vi "读MCDS参数设置.vi"() -> ()   [LabVIEW 2010]
uses:
  <vilib>/Utility/file.llb/Write To Spreadsheet File (string).vi
  GlobalVariable.vi
panel:
  out "选定曲线信息":string[](array[string])
  in  "曲线显示开关":bool[](array[boolean])
  in  "地址":sgl[][](array[numeric])
  in  "附加10点地址":i32=4
  in  "TCP 端口":i32=4
  in  "报警限值":sgl
  in  "报警延时":i32
  in  "报警点地址":i32
  in  "写寄存器数量":i32=4
  in  "写寄存器开始地址":i32=4
  in  "读寄存器数量":i32=4
  in  "读寄存器开始地址":i32=4
  in  "下段文件浏览":bool
  in  "上段文件浏览":bool
  in  "TCP IP地址":string
  in  "USB虚拟串口":string
  in  "取消修改":bool caption="Cancel Button"
  in  "保存修改":bool
  # "读取MCDS网络参数设置"
  # "坐标MAX"
  # "坐标MIN"
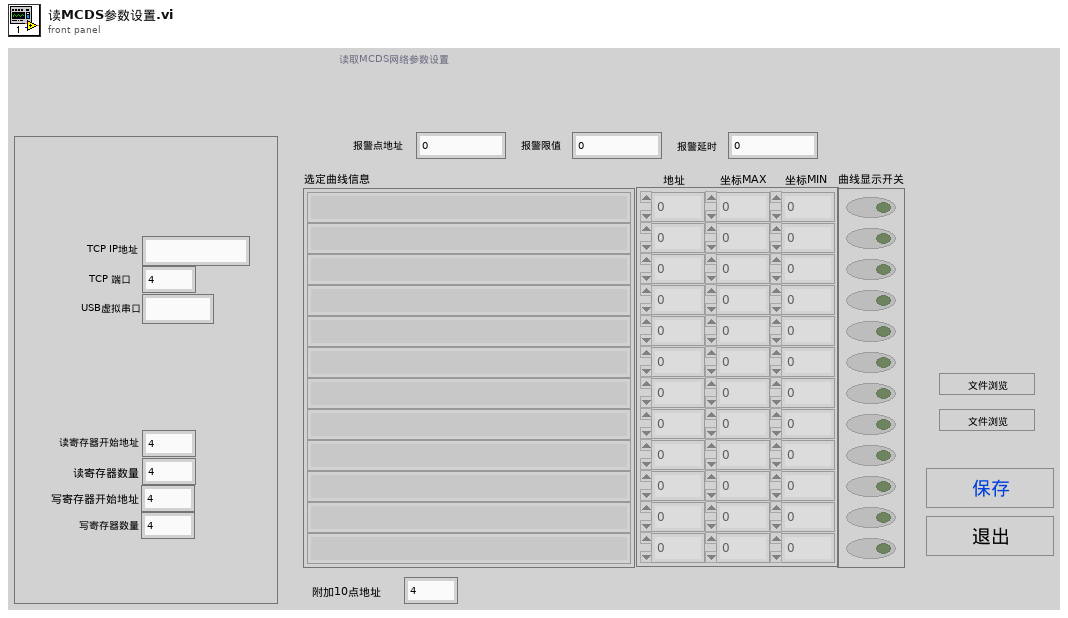
[diagram p1: front panel]
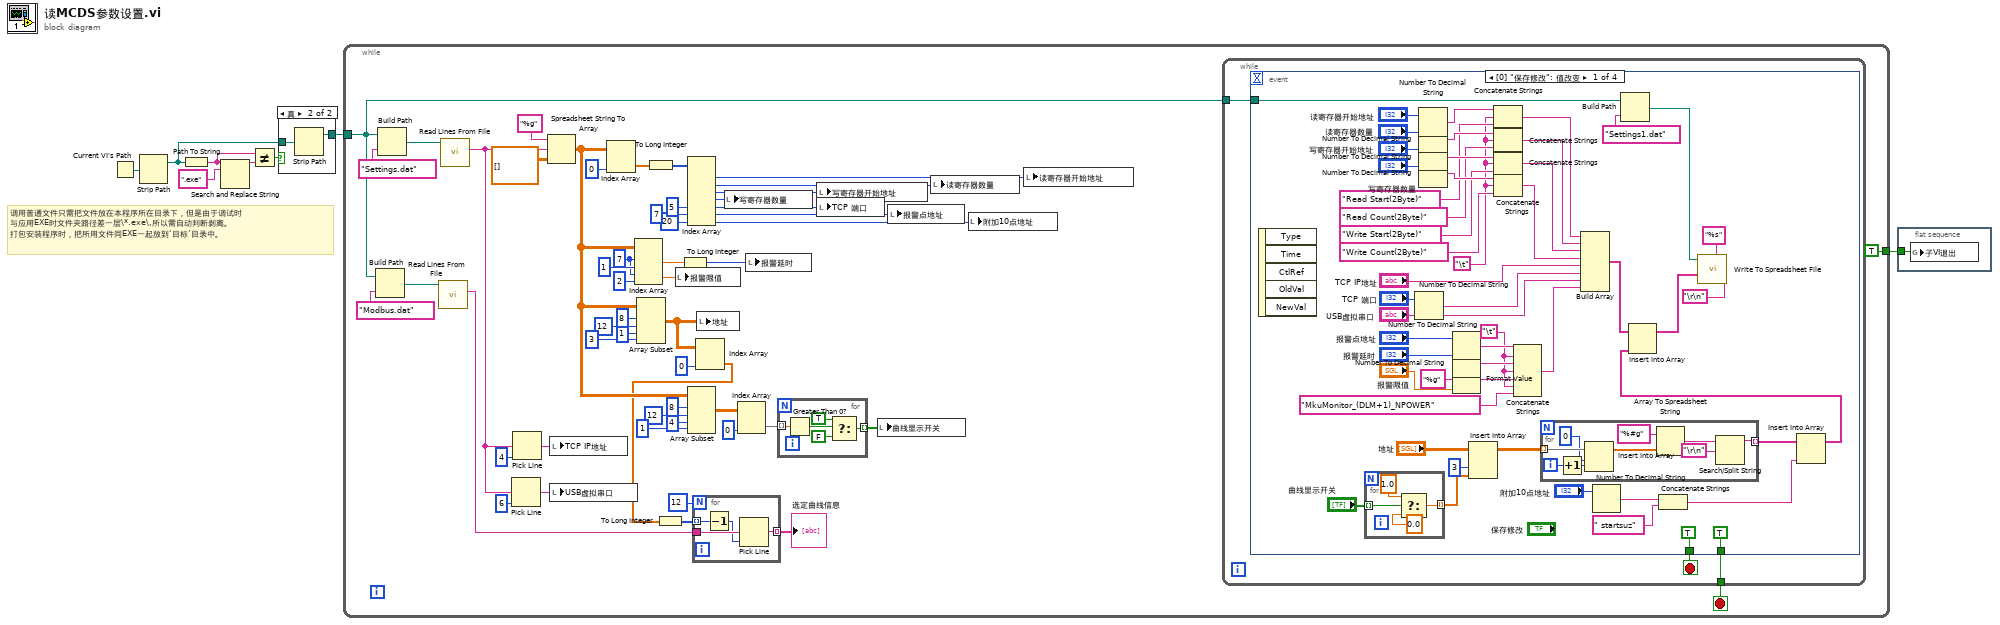
[diagram p0: block diagram]
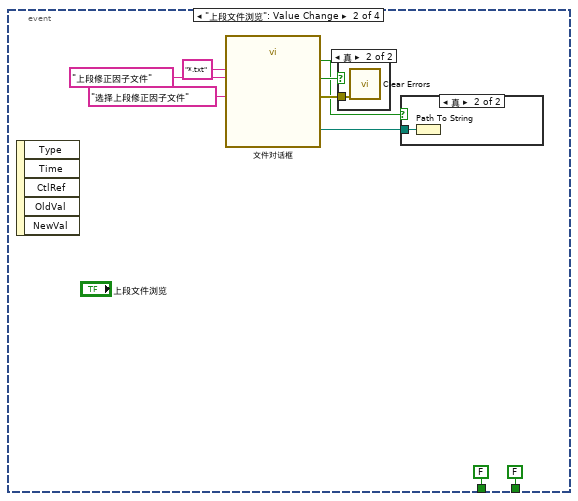
[diagram p3: hidden frame]
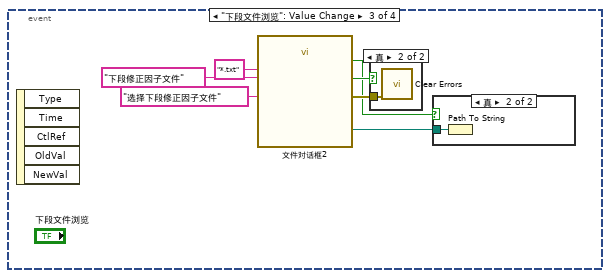
[diagram p6: hidden frame]
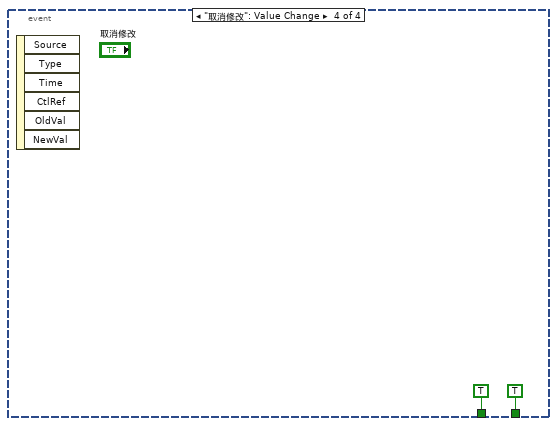
[diagram p9: hidden frame]
diagram:
  # "调用普通文件只需把文件放在本程序所在目录下，但是由于调试时\n与应用EXE时文件夹路径差一层\\*.exe\\,所以需自动判断剥离。\n打包安装程序时，把所用文件同EXE一起放到‘目标’目录中。"
  n1 = Current VI's Path() -> (path=w3:path)
  n2 = Strip Path(path=w3) -> (stripped path=w8:path)  [unwired: 1 out]
  n3 = Path To String(path=w8) -> (string=w6:string)
  n4 = Search and Replace String(input string=w6, search string=".exe" ("搜索字符串")) -> (result string=w5:string)  [unwired: 6 in, 3 out]
  n5 = Not Equal?(x=w6, y=w5) -> (x != y?=w7:bool)
  n6 = case shown="真" w7 {
    tunnel: w8 -> [w9 w11]
    tunnel: [w9 w10] -> w2
    frame False {
    }
    frame True {
      n7 = Strip Path(path=w11) -> (stripped path=w10:path)  [unwired: 1 out]
    }
  }
  n8 = while {
    tunnel: w2 -> [w12]
    tunnel: [TRUE ("子VI退出")] -> w1
    stop <- w63 stop-if-true
    w39 = 7 ("索引 (行)")
    n9 = Build Path(base path=w12, name or relative path="Modbus.dat") -> (appended path=w20:path)
    n10 = Build Path(base path=w12, name or relative path="Settings.dat") -> (appended path=w61:path)
    n11 = call <vilib>:"Read Lines From File.vi"("file path (dialog if empty)"=w20) -> ("line string"=w19:string)  [unwired: 5 in, 3 out]
    n12 = call <vilib>:"Read Lines From File.vi"("file path (dialog if empty)"=w61) -> ("line string"=w52:string)  [unwired: 5 in, 3 out]
    n13 = Pick Line ("选行并添加至字符串")(multi-line string=w52, line index=6 ("行索引")) -> (output string=w51:string)  [unwired: 1 in]
    n14 = Pick Line ("选行并添加至字符串")(multi-line string=w52, line index=4 ("行索引")) -> (output string=w54:string)  [unwired: 1 in]
    n15 = Spreadsheet String To Array ("电子表格字符串至数组转换")(format string="%g" ("format (%.3f)"), spreadsheet string=w52, array type (2D Dbl)=sgl[][] [] ("数组类型(2D Dbl)")) -> (array=w26:sgl[][])  [unwired: 1 in]
    n16 = local write "TCP IP地址"(w54) -> ()
    n17 = local write "USB虚拟串口"(w51) -> ()
    n18 = Index Array(array=w26, index (col)=0 ("禁用的索引 (列)")) -> (element=w48:sgl[])  [unwired: 1 in]
    n19 = Index Array(array=w26, index (row) #1=w39, index (col) #1=1 ("禁用的索引 (列)"), index (row) #2=w39, index (col) #2=2 ("禁用的索引 (列)")) -> (element #1=w36:sgl, element #2=w37:sgl)
    n20 = Array Subset(array=w26, index (row)=8 ("索引"), length (row)=12 ("长度"), index (col)=1 ("索引"), length (col)=3 ("长度")) -> (w13:sgl[][])
    n21 = To Long Integer(number=w48) -> (32bit integer=w47:i32[])
    n22 = local write "报警限值"(w37) -> ()
    n23 = To Long Integer(number=w36) -> (32bit integer=w35:i32)
    n24 = Index Array(array=w47, index #5=5 ("索引"), index #6=7 ("索引"), index #7=20 ("索引")) -> (element #1=w59:i32, element #2=w58:i32, element #3=w57:i32, element #4=w56:i32, element #5=w45:i32, element #6=w43:i32, element #7=w41:i32)  [unwired: 4 in]
    n25 = Array Subset(array=w26, index (row)=8 ("索引"), length (row)=12 ("长度"), index (col)=4 ("索引"), length (col)=1 ("长度")) -> (w25:sgl[][])
    n26 = Index Array(array=w13, index (col)=0 ("禁用的索引 (列)")) -> (element=w15:sgl[])  [unwired: 1 in]
    n27 = To Long Integer(number=w15) -> (32bit integer=w14:i32[])
    n28 = for {
      N: 12 -> [_]
      tunnel: w19 -> [w68]
      tunnel: [w67] -> w18 mode=indexing
      tunnel: w14 -> [w66] mode=indexing
      n29 = Decrement(x=w66) -> (x-1=w65:i32)
      n30 = Pick Line ("选行并添加至字符串")(multi-line string=w68, line index=w65) -> (output string=w67:string)  [unwired: 1 in]
    }
    "选定曲线信息" <- w18
    n31 = local write "地址"(w13) -> ()
    n32 = local write "写寄存器数量"(w56) -> ()
    n33 = Index Array(array=w25, index (col)=0 ("禁用的索引 (列)")) -> (element=w23:sgl[])  [unwired: 1 in]
    n34 = local write "报警延时"(w35) -> ()
    n35 = for {
      tunnel: w23 -> [w73] mode=indexing
      tunnel: [w69] -> w22 mode=indexing
      n36 = Greater Than 0?(x=w73) -> (x > 0?=w72:bool)
      n37 = Select(t=TRUE, s=w72, f=FALSE ("x > 0?")) -> (s? t:f=w69:bool)
    }
    n38 = local write "写寄存器开始地址"(w57) -> ()
    n39 = local write "TCP 端口"(w45) -> ()
    n40 = local write "曲线显示开关"(w22) -> ()
    n41 = local write "报警点地址"(w43) -> ()
    n42 = local write "读寄存器数量"(w58) -> ()
    n43 = local write "附加10点地址"(w41) -> ()
    n44 = local write "读寄存器开始地址"(w59) -> ()
    n45 = while {
      tunnel: [w76] -> w63
      tunnel: w12 -> [w75]
      stop <- w74 stop-if-true
      n46 = event shown="[0] \"保存修改\": 值改变" {
        selector: _ -> [_ _ _ _]
        dyn-events: _ -> [_ _ _ _]
        timeout: _ -> [_ _ _ _]
        tunnel: [TRUE FALSE _ TRUE] -> w74
        tunnel: w75 -> [w103 _ _ _]
        tunnel: [TRUE FALSE _ TRUE] -> w76
        event "保存修改": Value Change {
          w98 = "\t"
          w113 = "\t"
          n47 = event-data() -> ()  [unwired: 1 in, 5 out]
          n48 = for {
            tunnel: "曲线显示开关" -> [w131] mode=indexing
            tunnel: [w128] -> w78 mode=indexing
            n49 = Select(t=sgl 1.0 ("报警点地址"), s=w131, f=sgl 0.0 ("报警点地址")) -> (s? t:f=w128:sgl)
          }
          n50 = Number To Decimal String(number="TCP 端口") -> (decimal integer string=w92:string)  [unwired: 1 in]
          n51 = Number To Decimal String(number="读寄存器开始地址") -> (decimal integer string=w121:string)  [unwired: 1 in]
          n52 = Number To Decimal String(number="读寄存器数量") -> (decimal integer string=w120:string)  [unwired: 1 in]
          n53 = Number To Decimal String(number="写寄存器开始地址") -> (decimal integer string=w119:string)  [unwired: 1 in]
          n54 = Number To Decimal String(number="写寄存器数量") -> (decimal integer string=w118:string)  [unwired: 1 in]
          n55 = Number To Decimal String(number="报警点地址") -> (decimal integer string=w102:string)  [unwired: 1 in]
          n56 = Number To Decimal String(number="报警延时") -> (decimal integer string=w101:string)  [unwired: 1 in]
          n57 = Format Value(format string="%g" ("format (%.3f)"), value (0)="报警限值") -> (output string=w100:string)  [unwired: 1 in]
          n58 = Insert Into Array(array="地址", index (col)=3 ("禁用的索引 (列)"), new element=w78) -> (w79:sgl[][])  [unwired: 1 in]
          n59 = Concatenate Strings(w121, w113, "Read Start(2Byte)" ("十进制整型字符串")) -> (w97:string)
          n60 = Concatenate Strings(w120, w113, "Read Count(2Byte)" ("十进制整型字符串")) -> (w96:string)
          n61 = Concatenate Strings(w119, w113, "Write Start(2Byte)" ("十进制整型字符串")) -> (w95:string)
          n62 = Concatenate Strings(w118, w113, "Write Count(2Byte)" ("十进制整型字符串")) -> (w94:string)
          n63 = Concatenate Strings(w102, w98, w101, w98, w100, w98, "MkuMonitor_(DLM+1)_NPOWER" ("十进制整型字符串")) -> (w90:string)
          n64 = for {
            tunnel: w79 -> [w139] mode=indexing
            tunnel: [w132] -> w88 mode=indexing
            i -> [w138]
            n65 = Increment(x=w138) -> (x+1=w137:i32)
            n66 = Insert Into Array(array=w139, index=0 ("索引"), new element=w137) -> (w135:sgl[])
            n67 = Array To Spreadsheet String(array=w135, 3:"%#g" ("format string")) -> (spreadsheet string=w134:string)  [unwired: 1 in]
            n68 = Search/Split String(string=w134, search string/char (-)="\r\n") -> (substring before match=w132:string)  [unwired: 1 in, 2 out]
          }
          n69 = Build Array(w97, w96, w95, w94, "TCP IP地址", w92, "USB虚拟串口", w90) -> (w89:string[])
          n70 = Number To Decimal String(number="附加10点地址") -> (decimal integer string=w106:string)  [unwired: 1 in]
          n71 = Build Path(base path=w103, name or relative path="Settings1.dat") -> (appended path=w85:path)
          n72 = Concatenate Strings(w106, " startsuz" ("字符串")) -> (w86:string)
          n73 = Insert Into Array(array=w88, new element=w86) -> (w87:string[])  [unwired: 1 in]
          n74 = Insert Into Array(array=w89, new element=w87) -> (w84:string[])  [unwired: 1 in]
          n75 = call-poly <vilib>:"Write To Spreadsheet File.vi"("delimiter (\\t)"="\r\n", "format (%s)"="%s", "1D data"=w84, "file path (dialog if empty)"=w85) -> ()  [unwired: 4 in, 1 out]
        }
        event "上段文件浏览": Value Change {
          n76 = event-data() -> ()  [unwired: 1 in, 5 out]
          n77 = call "文件对话框"("prompt"="选择上段修正因子文件", "pattern (all files)"="*.txt", "pattern label"="上段修正因子文件") -> ("selected path"=w141:path, "exists"=w142:bool, "cancelled"=w143:bool, "error out"=w144:errorcluster)  [unwired: 9 in]
          n78 = case shown="真" w143 {
            tunnel: w144 -> [_ w151]
            frame False {
            }
            frame True {
              n79 = call <vilib>:"Clear Errors.vi"("error in (no error)"=w151) -> ()  [unwired: 6 in, 1 out]
            }
          }
          n80 = case shown="真" w142 {
            tunnel: w141 -> [_ w150]
            frame False {
            }
            frame True {
              n81 = Path To String(path=w150) -> ()  [unwired: 1 out]
            }
          }
        }
        event "下段文件浏览": Value Change {
          n82 = event-data() -> ()  [unwired: 1 in, 5 out]
          n83 = call "文件对话框2"("prompt"="选择下段修正因子文件", "pattern (all files)"="*.txt", "pattern label"="下段修正因子文件") -> ("selected path"=w152:path, "exists"=w153:bool, "cancelled"=w154:bool, "error out"=w155:errorcluster)  [unwired: 9 in]
          n84 = case shown="真" w154 {
            tunnel: w155 -> [_ w160]
            frame False {
            }
            frame True {
              n85 = call <vilib>:"Clear Errors.vi"("error in (no error)"=w160) -> ()  [unwired: 6 in, 1 out]
            }
          }
          n86 = case shown="真" w153 {
            tunnel: w152 -> [_ w159]
            frame False {
            }
            frame True {
              n87 = Path To String(path=w159) -> ()  [unwired: 1 out]
            }
          }
        }
        event "取消修改": Value Change {
          n88 = event-data() -> ()  [unwired: 1 in, 6 out]
        }
      }
    }
  }
  n89 = flat-sequence {
    tunnel: w1 -> [w163]
    frame #0 {
      n90 = global write "GlobalVariable.vi" "子VI退出"(w163) -> ()
    }
  }
